vi "NumberOFAI.vi"(0 "Refnum in":refnum<k21>, 2 "error in (no error)":errorcluster) -> (14 "Refnum out":refnum<k21>, 15 "Numeric":i32, 16 "error out":errorcluster)   [LabVIEW 2011]
uses:
  C:/Program Files/National Instruments/LabVIEW 2011/resource/objmgr/daqmx.rc
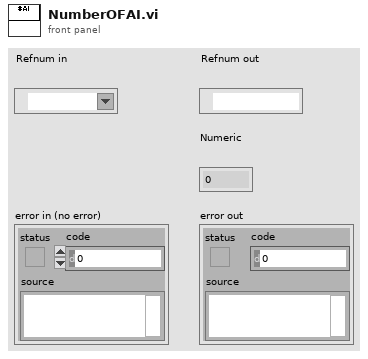
[diagram p1: front panel]
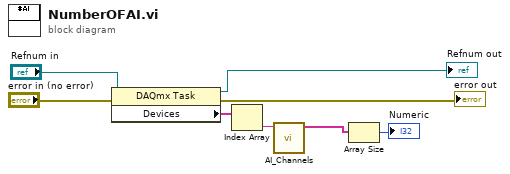
[diagram p0: block diagram]
diagram:
  n1 = property class="DAQmx Task"(reference="Refnum in", error in="error in (no error)") -> (reference out=→"Refnum out":refnum<k21>, error out=→"error out":errorcluster, "Devices"=w2:tag[])
  n2 = Index Array(array=w2) -> (element=w1:tag)  [unwired: 1 in]
  n3 = call "AI_Channels.vi"("DAQmx Device Name"=w1) -> ("Array"=w3:tag[])  [unwired: 9 in, 1 out]
  n4 = Array Size(array=w3) -> (size(s)=→"Numeric":i32)
